vi "AMC QMH Template (Windows CE).vi"() -> ()   [LabVIEW 2017]
doc: "Use this template to create a Touch Panel VI."
panel:
  out "Status":string
  in  "State Variables":cluster{"CurrentFile":path}
  in  "Exit":bool
  in  "Process":bool
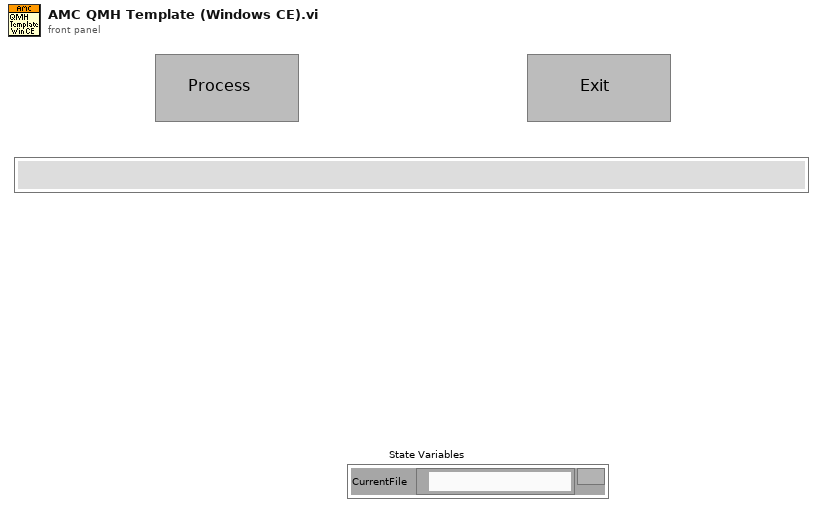
[diagram p1: front panel]
types:
  T1 = typedef "amc_Message Queue.ctl" = refnum<queue>
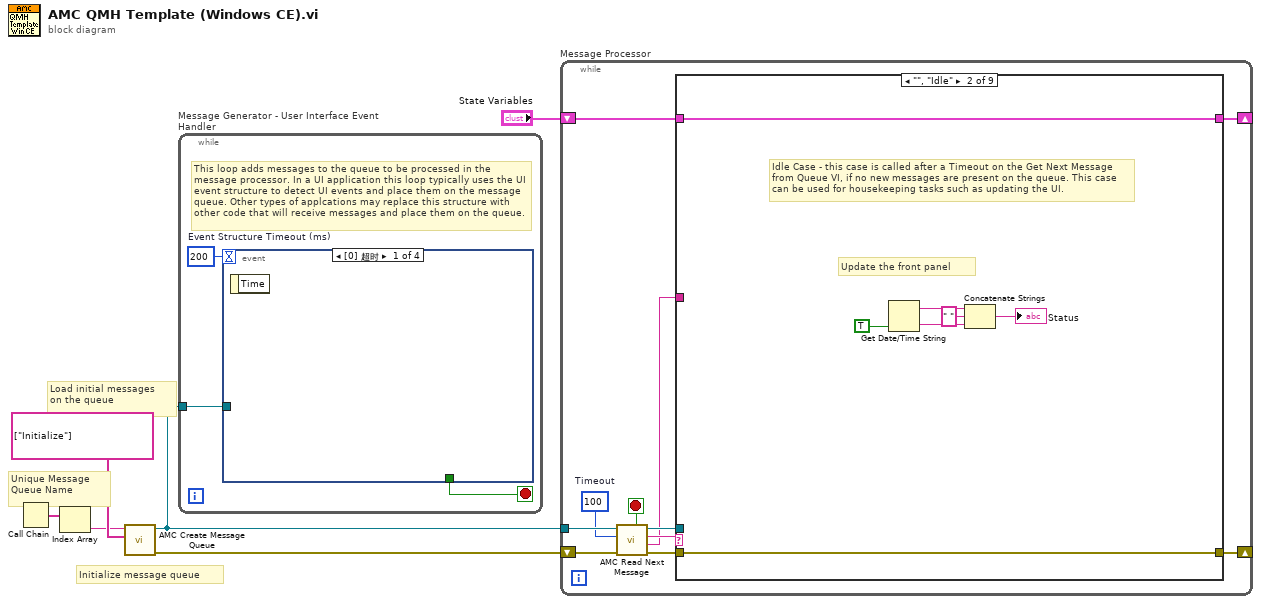
[diagram p0: block diagram]
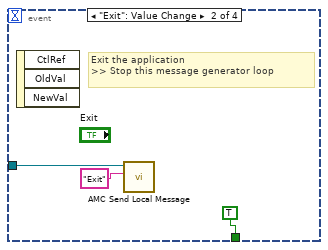
[diagram p2: hidden frame]
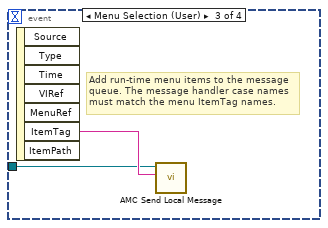
[diagram p3: hidden frame]
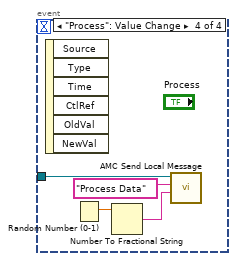
[diagram p4: hidden frame]
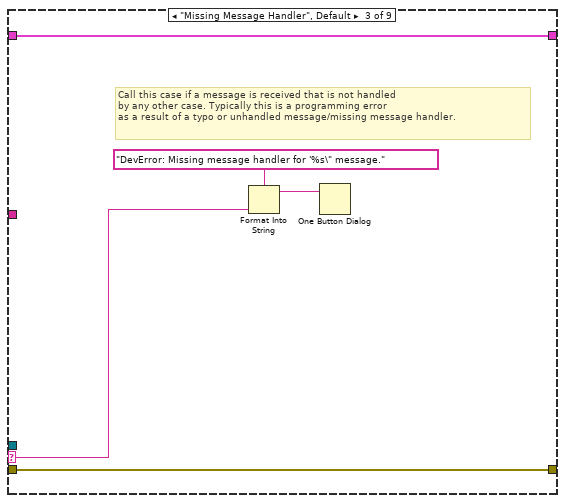
[diagram p6: hidden frame]
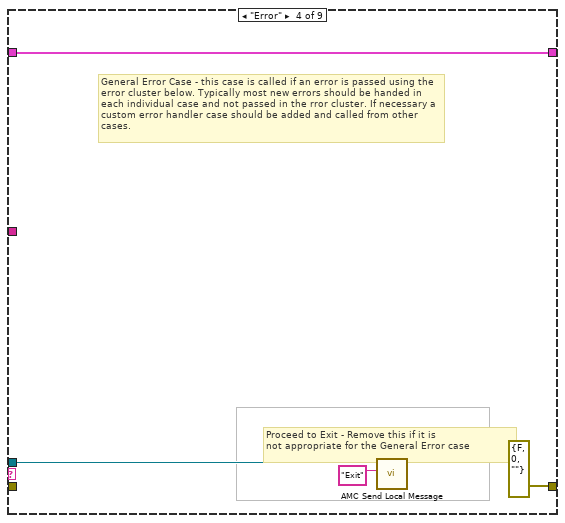
[diagram p7: hidden frame]
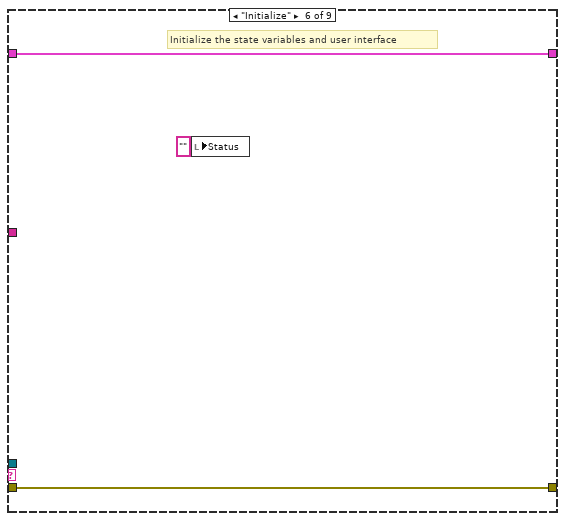
[diagram p9: hidden frame]
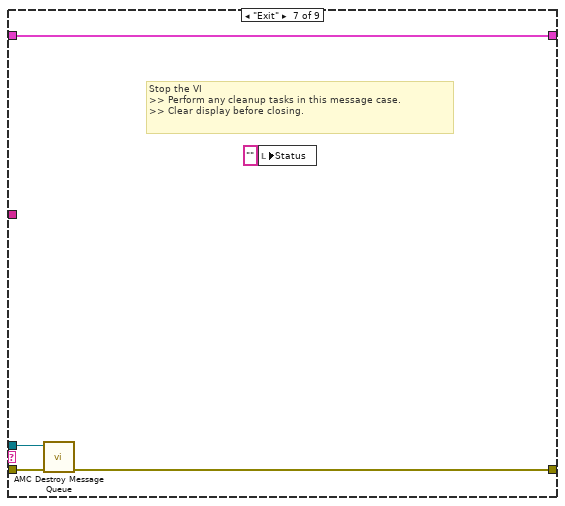
[diagram p10: hidden frame]
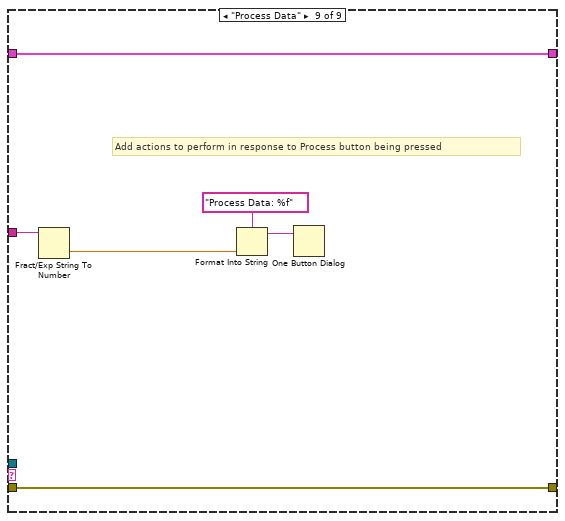
[diagram p12: hidden frame]
diagram:
  # "Initialize message queue"
  # "Unique Message\nQueue Name"
  # "Load initial messages\non the queue"
  n1 = Call Chain() -> (call chain=w2:string[])
  n2 = Index Array(array=w2) -> (element=w1:string)  [unwired: 1 in]
  n3 = call "AMC Create Message Queue.vi"("Initial Message Names"=string[] ["Initialize"], "Message Queue Name"=w1) -> ("error out"=w4:errorcluster, "Message Queue out"=w5:T1)  [unwired: 2 in, 6 out]
  n4 = while "Message Generator - User Interface Event Handler" {
    tunnel: w5 -> [w7]
    stop <- w8 stop-if-true
    w9 = 200  # Event Structure Timeout (ms)
    # "This loop adds messages to the queue to be processed in the message processor. In a UI application this loop typically uses the UI event structure to detect UI events and place them on the message queue. Other types of applcations may replace this structure with other code that will receive messages and place them on the queue."
    n5 = event shown="[0] 超时" {
      selector: _ -> [_ _ _ _]
      dyn-events: _ -> [_ _ _ _]
      timeout: w9 -> [_ _ _ _]
      tunnel: [_ TRUE ("Discard?") _ _] -> w8
      tunnel: w7 -> [_ w10 w13 w18]
      event Timeout {
        n6 = event-data() -> ()  [unwired: 2 out]
      }
      event "Exit": Value Change {
        # "Exit the application\n>> Stop this message generator loop"
        n7 = event-data() -> ()  [unwired: 4 out]
        n8 = call "AMC Send Local Message.vi"("Message Name"="Exit", "Message Queue in"=w10) -> ()  [unwired: 4 in, 6 out]
      }
      event Menu Selection (User) {
        # "Add run-time menu items to the message\nqueue. The message handler case names must match the menu ItemTag names."
        n9 = event-data() -> ("ItemTag"=w14:string)  [unwired: 7 out]
        n10 = call "AMC Send Local Message.vi"("Message Name"=w14, "Message Queue in"=w13) -> ()  [unwired: 4 in, 6 out]
      }
      event "Process": Value Change {
        n11 = event-data() -> ()  [unwired: 7 out]
        n12 = Random Number (0-1)() -> (number: 0 to 1=w15:dbl)
        n13 = Number To Fractional String(number=w15) -> (F-format string=w16:string)  [unwired: 3 out]
        n14 = call "AMC Send Local Message.vi"("Message Value"=w16, "Message Name"="Process Data", "Message Queue in"=w18) -> ()  [unwired: 3 in, 6 out]
      }
    }
  }
  n15 = while "Message Processor" {
    shift-left: w4 -> [w23]
    shift-right: [w27] -> _
    tunnel: w5 -> [w24]
    shift-left: "State Variables" -> [w29]
    shift-right: [w28] -> _
    stop <- w26 stop-if-true
    w21 = 100  # Timeout
    n16 = call "AMC Read Next Message.vi"("error in (no error)"=w23, "timeout (1ms)"=w21, "Message Queue in"=w24) -> ("error out"=w22:errorcluster, "Message Value"=w19:string, "Message Name"=w20:string, "Message Queue out"=w25:T1, "Exit Process"=w26:bool)  [unwired: 1 in, 3 out]
    n17 = case shown="\"\", \"Idle\"" w20 {
      selector: w20 -> [_ _ w41 _ _ _ _ _ _]
      tunnel: [w31 w38 w43 w47 w49 w52 w57 w59 w64] -> w28
      tunnel: w29 -> [w31 w38 w43 w47 w49 w52 w57 w59 w64]
      tunnel: w25 -> [_ _ _ w45 _ _ w54 _ _]
      tunnel: w22 -> [w30 w37 w42 _ w48 w51 w55 w58 w65]
      tunnel: [w30 w37 w42 errorcluster {"status"=FALSE, "code"=0, "source"=""} ("error out") w48 w51 w53 w58 w65] -> w27
      tunnel: w19 -> [_ _ _ _ _ _ _ _ w63]
      frame "---------- Framework Operations ----------" {
        # "Dummy case to add a seperator in the Case Structure menu"
      }
      frame "", "Idle" {
        # "Update the front panel"
        # "Idle Case - this case is called after a Timeout on the Get Next Message from Queue VI, if no new messages are present on the queue. This case can be used for housekeeping tasks such as updating the UI."
        n18 = Get Date/Time String(want seconds? (F)=TRUE) -> (date string=w36:string, time string=w35:string)  [unwired: 2 out]
        n19 = Concatenate Strings(w36, " " ("string"), w35) -> (→"Status":string)
      }
      frame "Missing Message Handler", Default {
        # "Call this case if a message is received that is not handled \nby any other case. Typically this is a programming error\nas a result of a typo or unhandled message/missing message handler."
        n20 = Format Into String(format string="DevError: Missing message handler for '%s\" message." ("message"), w41) -> (resulting string=w39:string)  [unwired: 2 in, 1 out]
        n21 = One Button Dialog(message=w39) -> ()  [unwired: 2 out]
      }
      frame "Error" {
        # "Proceed to Exit - Remove this if it is\nnot appropriate for the General Error case"
        # "General Error Case - this case is called if an error is passed using the error cluster below. Typically most new errors should be handed in each individual case and not passed in the rror cluster. If necessary a custom error handler case should be added and called from other cases."
        n22 = call "AMC Send Local Message.vi"("Message Name"="Exit", "Message Queue in"=w45) -> ()  [unwired: 4 in, 6 out]
      }
      frame "---------- Generic Operations ----------" {
        # "Dummy case to add a seperator in the Case Structure menu"
      }
      frame "Initialize" {
        # "Initialize the state variables and user interface"
        n23 = local write "Status"("" ("Status")) -> ()
      }
      frame "Exit" {
        # "Stop the VI\n>> Perform any cleanup tasks in this message case.\n>> Clear display before closing."
        n24 = call "AMC Destroy Message Queue.vi"("error in (no error)"=w55, "Message Queue in"=w54) -> ("error out"=w53:errorcluster)  [unwired: 9 out]
        n25 = local write "Status"("" ("Status")) -> ()
      }
      frame "---------- Application Operations ----------" {
        # "Dummy case to add a seperator in the Case Structure menu"
      }
      frame "Process Data" {
        # "Add actions to perform in response to Process button being pressed"
        n26 = Fract/Exp String To Number(string=w63) -> (number=w62:dbl)  [unwired: 4 out]
        n27 = Format Into String(format string="Process Data: %f" ("message"), w62) -> (resulting string=w60:string)  [unwired: 2 in, 1 out]
        n28 = One Button Dialog(message=w60) -> ()  [unwired: 2 out]
      }
    }
  }
